vi "s-5 girilen tek sayıları tespit edip diziye yazdıran program 2018 19.vi"() -> ()   [LabVIEW 2014]
panel:
  out "Array 2":dbl[](array[numeric])
  in  "ilk":dbl[](array[numeric])
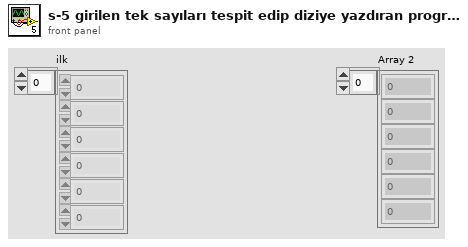
[diagram p1: front panel]
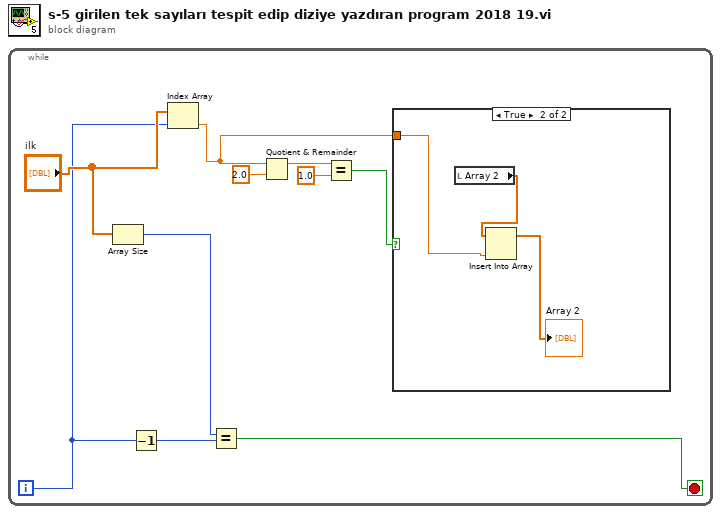
[diagram p0: block diagram]
diagram:
  n1 = while {
    i -> [w8]
    stop <- w3 stop-if-true
    n2 = Array Size(array="ilk") -> (size(s)=w6:i32)
    n3 = Decrement(x=w8) -> (x-1=w7:i32)
    n4 = Index Array(array="ilk", index=w8) -> (element=w1:dbl)
    n5 = Equal?(x=w6, y=w7) -> (x = y?=w3:bool)
    n6 = Quotient & Remainder(x=w1, y=2.0) -> (x-y*floor(x/y)=w5:dbl)  [unwired: 1 out]
    n7 = Equal?(x=w5, y=1.0) -> (x = y?=w2:bool)
    n8 = case shown="True" w2 {
      tunnel: w1 -> [_ w12]
      frame False {
      }
      frame True {
        n9 = local read "Array 2"() -> (w13:dbl[])
        n10 = Insert Into Array(array=w13, new element=w12) -> (→"Array 2":dbl[])  [unwired: 1 in]
      }
    }
  }
